vi "Calculate Particle Scores Port no Bottom Target.vi"(10 "Sorted Data":dbl[][](array[numeric])) -> (3 "Scores":T1[](array[typedef]))   [LabVIEW 2023]
doc: "Calculate scores based on the particle measurements. Calculated scores are for aspect ratio, area to convex hull area, and moment of inertia. These scores range between 0 and 100 and can be used to categorize particles as targets and non-targets."
uses:
  Target Fields.ctl
  <vilib>/Analysis/baseanly.llb/Mean (DBL).vi
  <vilib>/Analysis/NI_AALBase.lvlib
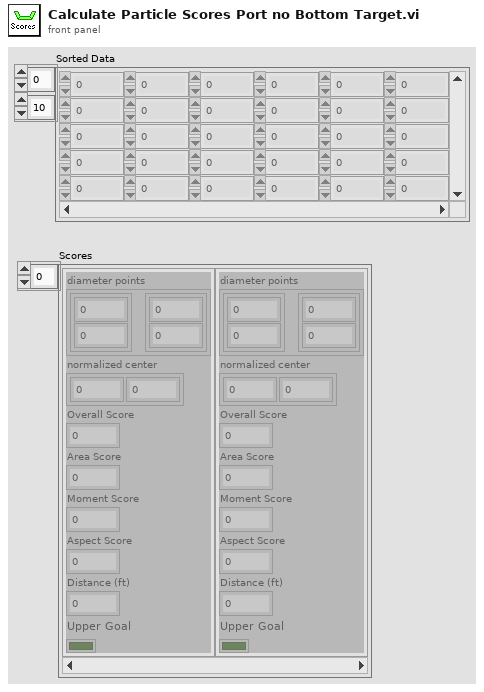
[diagram p1: front panel]
types:
  T1 = typedef "Target Fields.ctl" = cluster{"diameter points":cluster{"first point":cluster{"x":dbl, "y":dbl}, "projected point":cluster{"x":dbl, "y":dbl}}, "normalized center":cluster{"x":dbl, "y":dbl}, "Overall Score":dbl, "Area Score":dbl, "Moment Score":dbl, "Aspect Score":dbl, "Distance (ft)":dbl, "Upper Goal":bool}
  T2 = cluster{cluster{"Numeric":dbl, "Numeric":dbl}, cluster{"Numeric":dbl, "Numeric":dbl}}
  T3 = cluster{"first point":cluster{"x":dbl, "y":dbl}, "projected point":cluster{"x":dbl, "y":dbl}}
  T4 = cluster{cluster{"first point":cluster{"x":dbl, "y":dbl}, "projected point":cluster{"x":dbl, "y":dbl}}, "first point":cluster{"x":dbl, "y":dbl}, "mean":dbl, "Score":dbl, "Score":dbl, "Score":dbl, dbl, bool}
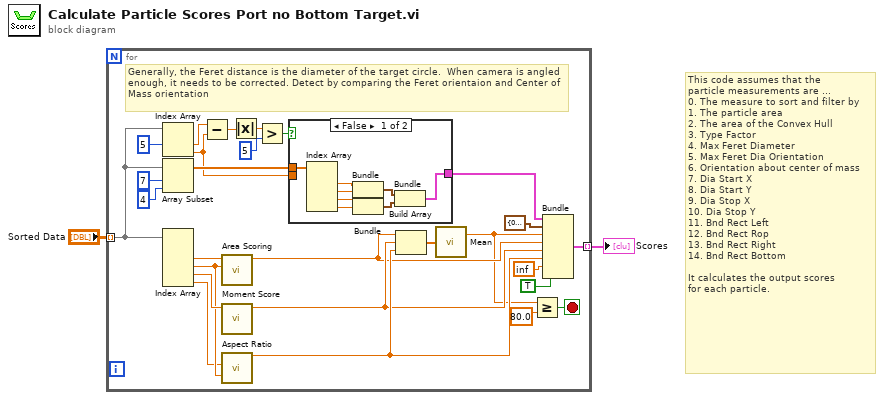
[diagram p0: block diagram]
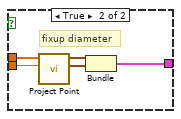
[diagram p2: hidden frame]
diagram:
  # "This code assumes that the\nparticle measurements are ...\n0. The measure to sort and filter by\n1. The particle area\n2. The area of the Convex Hull\n3. Type Factor\n4. Max Feret Diameter\n5. Max Feret Dia Orientation\n6. Orientation about center of mass\n7. Dia Start X\n8. Dia Start Y\n9. Dia Stop X\n10. Dia Stop Y\n11. Bnd Rect Left\n12. Bnd Rect Rop\n13. Bnd Rect Right\n14. Bnd Rect Bottom\n\nIt calculates the output scores\nfor each particle."
  n1 = for {
    tunnel: "Sorted Data" -> [w8] mode=indexing
    tunnel: [w3] -> w1 mode=indexing
    stop <- w5 stop-if-true
    # "Generally, the Feret distance is the diameter of the target circle.  When camera is angled enough, it needs to be corrected. Detect by comparing the Feret orientaion and Center of Mass orientation"
    n2 = Index Array(array=w8, index #1=5 ("index")) -> (element #1=w22:dbl, element #2=w17:dbl)  [unwired: 1 in]
    n3 = Array Subset(array=w8, index=7, length=4) -> (w18:dbl[])
    n4 = Index Array(array=w8) -> (element #2=w29:dbl, element #3=w27:dbl, element #4=w28:dbl, element #5=w26:dbl)  [unwired: 5 in, 1 out]
    n5 = Subtract(x=w22, y=w17) -> (x-y=w25:dbl)
    n6 = call "Area Scoring.vi"("Convex Hull Area"=w27, "Area"=w29) -> ("Score"=w12:dbl)  [unwired: 9 in]
    n7 = call "Moment Score.vi"("Moment Factor"=w28) -> ("Score"=w13:dbl)  [unwired: 10 in]
    n8 = call "Aspect Ratio.vi"("Diameter"=w26, "Convex Hull Area"=w27) -> ("Score"=w14:dbl)  [unwired: 9 in]
    n9 = Absolute Value(x=w25) -> (abs(x)=w23:dbl)
    n10 = Greater?(x=w23, y=5 ("length")) -> (0:w16:bool)
    n11 = case shown="False" w16 {
      tunnel: w18 -> [w35 w42]
      tunnel: w17 -> [_ w41]
      tunnel: [w30 w38] -> w11
      frame False {
        n12 = Index Array(array=w35) -> (element #1=w33:dbl, element #2=w34:dbl, element #3=w36:dbl, element #4=w37:dbl)  [unwired: 4 in]
        n13 = Bundle("Numeric"=w33, "Numeric"=w34) -> (w32:cluster{"Numeric":dbl, "Numeric":dbl})  [unwired: 1 in]
        n14 = Bundle("Numeric"=w36, "Numeric"=w37) -> (w31:cluster{"Numeric":dbl, "Numeric":dbl})  [unwired: 1 in]
        n15 = Bundle(w32, w31) -> (w30:T2)  [unwired: 1 in]
      }
      frame True {
        # "fixup diameter"
        n16 = call "Project Point.vi"("orientation (deg)"=w41, "coordinates"=w42) -> ("projected point"=w39:cluster{"x":dbl, "y":dbl}, "first point"=w40:cluster{"x":dbl, "y":dbl})  [unwired: 8 in]
        n17 = Bundle("first point"=w40, "projected point"=w39) -> (w38:T3)  [unwired: 1 in]
      }
    }
    n18 = Build Array(w12, w13, w14) -> (w4:dbl[])
    n19 = call-poly <vilib>:"Mean.vi"("X"=w4) -> ("mean"=w7:dbl)  [unwired: 1 out]
    n20 = Greater Or Equal?(x=w7, y=80.0) -> (x >= y?=w5:bool)
    n21 = Bundle(w11, "first point"=cluster{"x":dbl, "y":dbl} {"x"=0.0, "y"=0.0}, "mean"=w7, "Score"=w12, "Score"=w13, "Score"=w14, inf, TRUE) -> (w3:T4)  [unwired: 1 in]
  }
  "Scores" <- w1
